vi "SDSU_SetSampling.vi"(8 "error in":errorcluster, 10 "sampling type":string, 11 "fd":i32) -> (0 "error out":errorcluster, 2 "read value":i32, 3 "fd":i32)   [LabVIEW 2016]
uses:
  DBSHAND/private/vis/DatabaseHand_Element_Set(string).vi
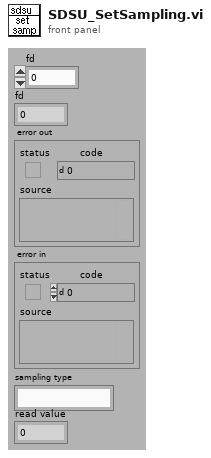
[diagram p1: front panel]
types:
  T1 = typedef "DatabaseHand_RefNum.ctl" = refnum<vi>
  T2 = typedef "DHE_Obs.ctl" = cluster{"observer":string, "obstype":string, "exptime":dbl, "coadds":i32, "fowler":i32, "nimages":i32, "display":bool, "autowrite":bool, "frames to write":cluster{"subs":bool, "reset":bool, "exposed":bool}, "frames to display":cluster{"subs":bool, "reset":bool, "exposed":bool}, "sur":i32}
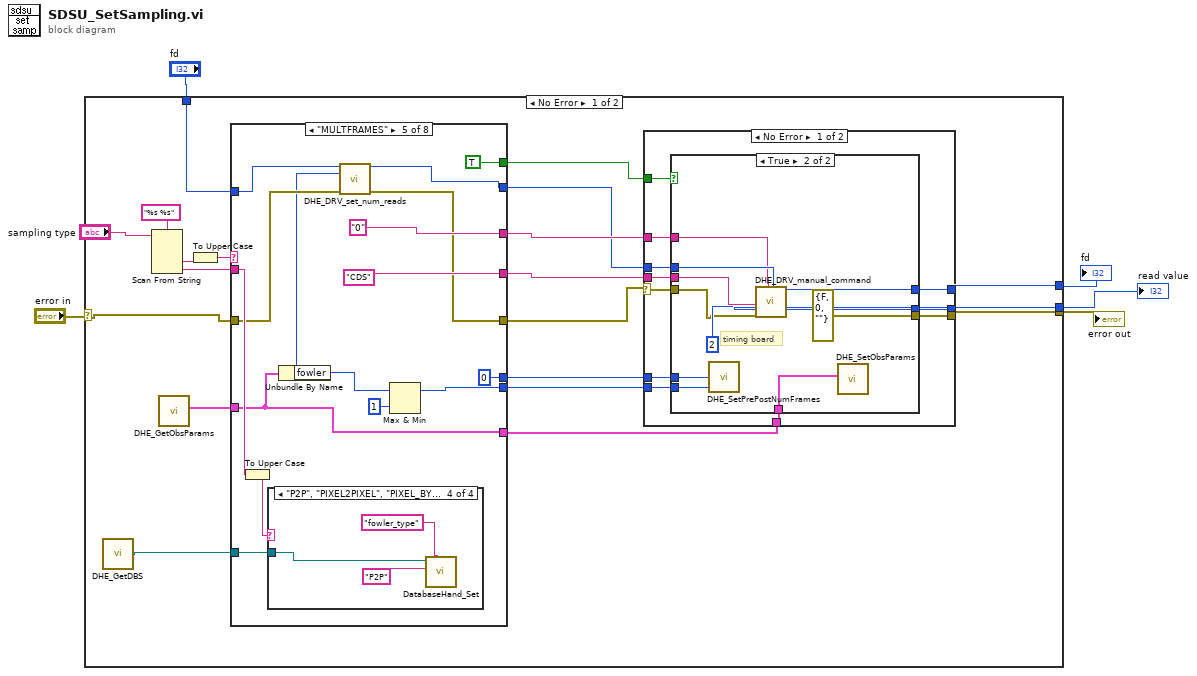
[diagram p0: block diagram]
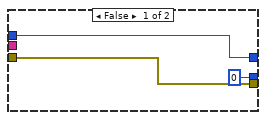
[diagram p2: hidden frame]
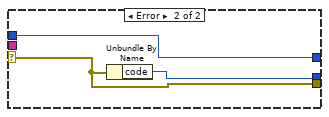
[diagram p3: hidden frame]
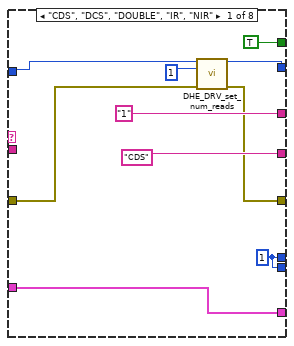
[diagram p4: hidden frame]
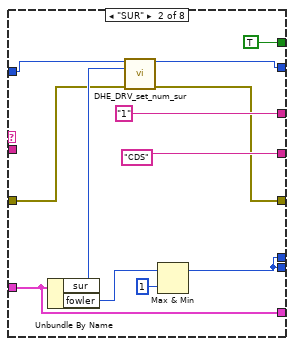
[diagram p5: hidden frame]
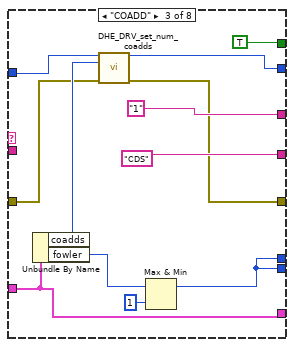
[diagram p6: hidden frame]
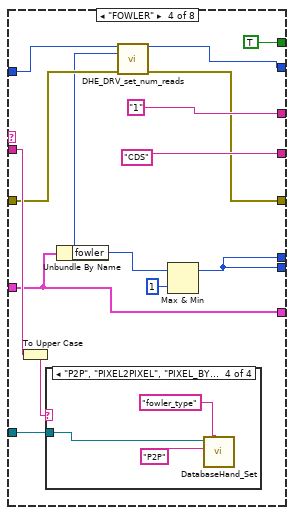
[diagram p7: hidden frame]
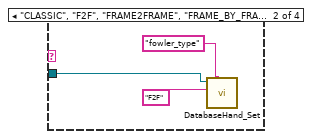
[diagram p9: hidden frame]
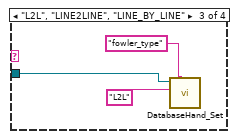
[diagram p10: hidden frame]
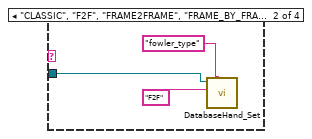
[diagram p12: hidden frame]
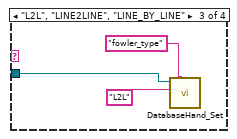
[diagram p13: hidden frame]
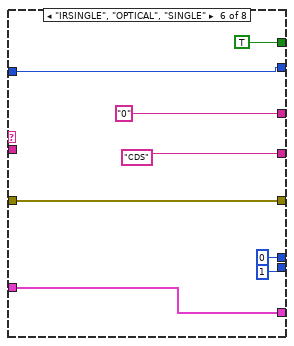
[diagram p14: hidden frame]
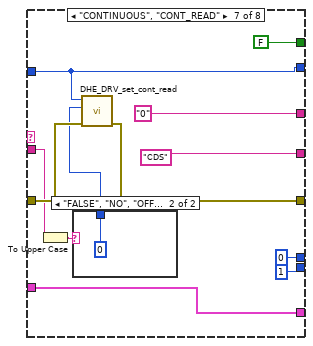
[diagram p15: hidden frame]
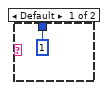
[diagram p16: hidden frame]
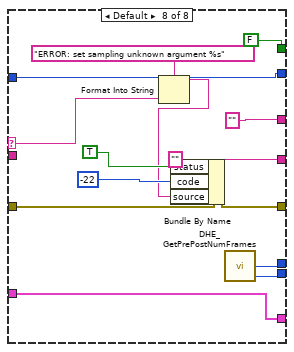
[diagram p17: hidden frame]
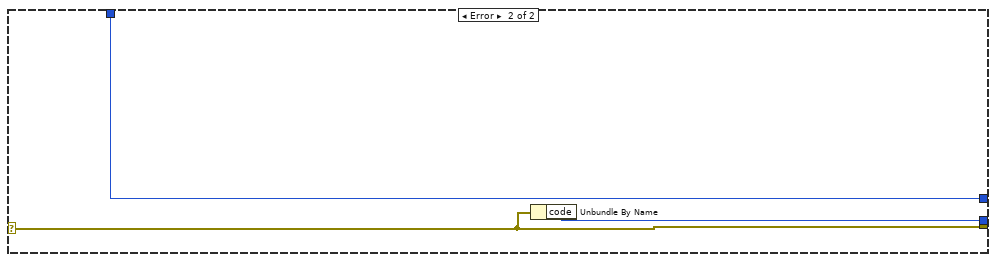
[diagram p18: hidden frame]
diagram:
  n1 = case shown="No Error" "error in" {
    selector: "error in" -> [w16 w172]
    tunnel: [w20 w173] -> w5
    tunnel: [w19 w172] -> w4
    tunnel: [w17 w171] -> w3
    tunnel: "fd" -> [w14 w173]
    frame No Error {
      n2 = call "DHE_GetDBS.vi"() -> ("DHE_DBSRef"=w6:T1)  [unwired: 9 out]
      n3 = Scan From String(format string="%s %s", input string="sampling type") -> (output 1=w24:string, output 2=w15:string)  [unwired: 2 in, 5 out]
      n4 = call "DHE_GetObsParams.vi"() -> ("DHE_OBS"=w13:T2)  [unwired: 11 out]
      n5 = To Upper Case(1:w24) -> (0:w23:string)
      n6 = case shown="\"MULTFRAMES\"" w23 {
        selector: w23 -> [_ _ _ _ _ _ _ w164]
        tunnel: w16 -> [w57 w69 w79 w95 w119 w141 w148 w169]
        tunnel: ["1" "1" "1" "1" "0" "0" "0" ""] -> w21
        tunnel: [w56 w68 w78 w94 w118 w141 w147 w168] -> w10
        tunnel: ["CDS" "CDS" "CDS" "CDS" "CDS" "CDS" "CDS" ""] -> w22
        tunnel: w15 -> [_ _ _ w99 w123 _ w145 _]
        tunnel: [w55 w64 w84 w96 0 ("DHE_PreExpose") 0 0 w159] -> w9
        tunnel: [w55 w64 w84 w96 w120 1 ("DHE_PreExpose") 1 ("DHE_PreExpose") w158] -> w8
        tunnel: w14 -> [w60 w73 w83 w93 w117 w137 w146 w161]
        tunnel: w13 -> [w61 w70 w81 w91 w115 w138 w151 w160]
        tunnel: [w61 w70 w81 w91 w115 w138 w151 w160] -> w12
        tunnel: [w59 w72 w82 w92 w116 w137 w146 w161] -> w11
        tunnel: [TRUE TRUE TRUE TRUE TRUE TRUE FALSE FALSE] -> w7
        tunnel: w6 -> [_ _ _ w88 w112 _ _ _]
        frame "CDS", "DCS", "DOUBLE", "IR", "NIR" {
          w55 = 1 ("DHE_PreExpose")
          n7 = call "DHE_DRV_set_num_reads.vi"("fd"=w60, "num_reads"=1, "error in (no error)"=w57) -> ("fd out"=w59:i32, "error out"=w56:errorcluster)  [unwired: 11 out]
        }
        frame "SUR" {
          n8 = Unbundle By Name(w70) -> ("sur"=w71:i32, "fowler"=w65:i32)
          n9 = call "DHE_DRV_set_num_sur.vi"("fd"=w73, "num_reads"=w71, "error in (no error)"=w69) -> ("fd out"=w72:i32, "error out"=w68:errorcluster)  [unwired: 11 out]
          n10 = Max & Min(x=w65, y=u16 1) -> (max(x,y)=w64:i32)  [unwired: 1 out]
        }
        frame "COADD" {
          n11 = Unbundle By Name(w81) -> ("coadds"=w80:i32, "fowler"=w77:i32)
          n12 = call "DHE_DRV_set_num_coadds.vi"("fd"=w83, "num_coadds"=w80, "error in (no error)"=w79) -> ("fd out"=w82:i32, "error out"=w78:errorcluster)  [unwired: 11 out]
          n13 = Max & Min(x=w77, y=u16 1) -> (max(x,y)=w84:i32)  [unwired: 1 out]
        }
        frame "FOWLER" {
          n14 = To Upper Case(1:w99) -> (0:w98:string)
          n15 = case shown="\"P2P\", \"PIXEL2PIXEL\", \"PIXEL_BY_PIXEL\"" w98 {
            tunnel: w88 -> [_ w102 w105 w108]
            frame Default {
            }
            frame "CLASSIC", "F2F", "FRAME2FRAME", "FRAME_BY_FRAME", "NORMAL" {
              n16 = call-poly "DatabaseHand_Set.vi"("name"="fowler_type", "value"="F2F", "Database RefNum in"=w102) -> ()  [unwired: 5 in, 4 out]
            }
            frame "L2L", "LINE2LINE", "LINE_BY_LINE" {
              n17 = call-poly "DatabaseHand_Set.vi"("name"="fowler_type", "value"="L2L", "Database RefNum in"=w105) -> ()  [unwired: 5 in, 4 out]
            }
            frame "P2P", "PIXEL2PIXEL", "PIXEL_BY_PIXEL" {
              n18 = call-poly "DatabaseHand_Set.vi"("name"="fowler_type", "value"="P2P", "Database RefNum in"=w108) -> ()  [unwired: 5 in, 4 out]
            }
          }
          n19 = Unbundle By Name(w91) -> ("fowler"=w90:i32)
          n20 = call "DHE_DRV_set_num_reads.vi"("fd"=w93, "num_reads"=w90, "error in (no error)"=w95) -> ("fd out"=w92:i32, "error out"=w94:errorcluster)  [unwired: 11 out]
          n21 = Max & Min(x=w90, y=u16 1) -> (max(x,y)=w96:i32)  [unwired: 1 out]
        }
        frame "MULTFRAMES" {
          n22 = To Upper Case(1:w123) -> (0:w122:string)
          n23 = case shown="\"P2P\", \"PIXEL2PIXEL\", \"PIXEL_BY_PIXEL\"" w122 {
            tunnel: w112 -> [_ w126 w129 w132]
            frame Default {
            }
            frame "CLASSIC", "F2F", "FRAME2FRAME", "FRAME_BY_FRAME", "NORMAL" {
              n24 = call-poly "DatabaseHand_Set.vi"("name"="fowler_type", "value"="F2F", "Database RefNum in"=w126) -> ()  [unwired: 5 in, 4 out]
            }
            frame "L2L", "LINE2LINE", "LINE_BY_LINE" {
              n25 = call-poly "DatabaseHand_Set.vi"("name"="fowler_type", "value"="L2L", "Database RefNum in"=w129) -> ()  [unwired: 5 in, 4 out]
            }
            frame "P2P", "PIXEL2PIXEL", "PIXEL_BY_PIXEL" {
              n26 = call-poly "DatabaseHand_Set.vi"("name"="fowler_type", "value"="P2P", "Database RefNum in"=w132) -> ()  [unwired: 5 in, 4 out]
            }
          }
          n27 = Unbundle By Name(w115) -> ("fowler"=w114:i32)
          n28 = call "DHE_DRV_set_num_reads.vi"("fd"=w117, "num_reads"=w114, "error in (no error)"=w119) -> ("fd out"=w116:i32, "error out"=w118:errorcluster)  [unwired: 11 out]
          n29 = Max & Min(x=w114, y=u16 1) -> (max(x,y)=w120:i32)  [unwired: 1 out]
        }
        frame "IRSINGLE", "OPTICAL", "SINGLE" {
        }
        frame "CONTINUOUS", "CONT_READ" {
          n30 = To Upper Case(1:w145) -> (0:w144:string)
          n31 = case shown="\"FALSE\", \"NO\", \"OFF\"" w144 {
            tunnel: [1 0] -> w143
            frame Default {
            }
            frame "FALSE", "NO", "OFF" {
            }
          }
          n32 = call "DHE_DRV_set_cont_read.vi"("error in (no error)"=w148, "arg1"=w143, "fd"=w146) -> ("error out"=w147:errorcluster)  [unwired: 8 out]
        }
        frame Default {
          n33 = Format Into String(format string="ERROR: set sampling unknown argument %s" ("source"), w164) -> (resulting string=w163:string)  [unwired: 2 in, 1 out]
          n34 = Bundle By Name(cluster=w169, "status"=TRUE, "code"=-22, "source"=w163) -> (w168:errorcluster)
          n35 = call "DHE_GetPrePostNumFrames.vi"() -> ("DHE_PreExpose"=w159:i32, "DHE_PostExpose"=w158:i32)  [unwired: 8 out]
        }
      }
      n36 = case shown="No Error" w10 {
        selector: w10 -> [w33 w52]
        tunnel: w11 -> [w36 w53]
        tunnel: [w35 w53] -> w20
        tunnel: [w34 w51] -> w17
        tunnel: [w30 w52] -> w19
        tunnel: w22 -> [w32 _]
        tunnel: w21 -> [w31 _]
        tunnel: w12 -> [w29 _]
        tunnel: w9 -> [w28 _]
        tunnel: w8 -> [w27 _]
        tunnel: w7 -> [w26 _]
        frame No Error {
          n37 = case shown="True" w26 {
            tunnel: w36 -> [w39 w50]
            tunnel: [w39 w49] -> w35
            tunnel: [0 ("error_code") w48] -> w34
            tunnel: w33 -> [w37 w46]
            tunnel: w32 -> [_ w45]
            tunnel: w31 -> [_ w44]
            tunnel: [w37 errorcluster {"status"=FALSE, "code"=0, "source"=""} ("error IO")] -> w30
            tunnel: w29 -> [_ w42]
            tunnel: w28 -> [_ w41]
            tunnel: w27 -> [_ w40]
            frame False {
            }
            frame True {
              # "timing board"
              n38 = call "DHE_SetPrePostNumFrames.vi"("DHE_PreExpose"=w41, "DHE_PostExpose"=w40) -> ()  [unwired: 8 out]
              n39 = call "DHE_DRV_manual_command.vi"("command"=w45, "short board_dest"=i16 2, "error in (no error)"=w46, "arg1"=w44, "fd"=w50) -> ("fd"=w49:i32, "error_code"=w48:i32)  [unwired: 4 in, 9 out]
              n40 = call "DHE_SetObsParams.vi"("DHE_OBS"=w42) -> ()  [unwired: 11 out]
            }
          }
        }
        frame Error {
          n41 = Unbundle By Name(w52) -> ("code"=w51:i32)
        }
      }
    }
    frame Error {
      n42 = Unbundle By Name(w172) -> ("code"=w171:i32)
    }
  }
  "fd" <- w5
  "error out" <- w4
  "read value" <- w3
